vi "Agilent VNA Set External Trigger Mode.vi"(7 "Agilent VNA":T2, 8 "error in (no error)":errorcluster, 10 "Ext. Trigger Mode":T1, 11 "VISA Resource Name":refnum<visa-resource-name>) -> (0 "error out":errorcluster, 2 "Previous Ext. Trigger Mode":T1, 3 "dup VISA Resource Name":refnum<visa-resource-name>)   [LabVIEW 2011]
doc: "This VI for the HP8753B Network Analyzers reads the stimulus values. Except when performing log sweeps and freq list sweeps, this VI uses the start and stop values and the number of points to calcuate the stimulus values."
uses:
  TypeDefs/Agilent VNA External Trigger Mode.ctl
  TypeDefs/Agilent VNA Instrument Info.ctl
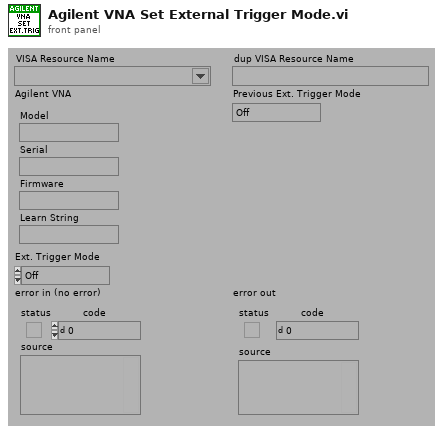
[diagram p1: front panel]
types:
  T1 = typedef "Agilent VNA External Trigger Mode.ctl" = enum16{"Off", "On Sweep", "On Point", "Manual On Point", "Internal", "External", "Bus"}
  T2 = typedef "Agilent VNA Instrument Info.ctl" = cluster{"Model":string, "Serial":string, "Firmware":string, "Learn String":string}
  T3 = typedef "Agilent VNA Model.ctl" = enum16{"Not Supported", "8510X", "8719X", "8720X", "8722X", "8753X", "ENA", "PNA", "Field Fox"}
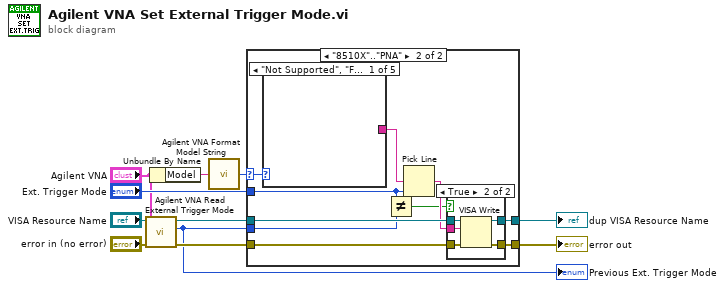
[diagram p0: block diagram]
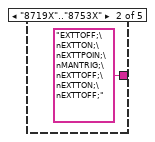
[diagram p3: hidden frame]
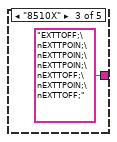
[diagram p4: hidden frame]
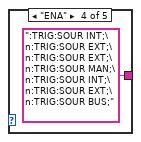
[diagram p5: hidden frame]
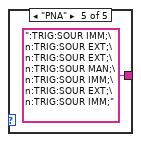
[diagram p6: hidden frame]
diagram:
  n1 = call "Agilent VNA Read External Trigger Mode.vi"("Agilent VNA"="Agilent VNA", "error in (no error)"="error in (no error)", "VISA Resource Name"="VISA Resource Name") -> ("error out"=w6:errorcluster, "Ext. Trigger Mode"=w4:T1, "dup VISA Resource Name"=w5:refnum<visa-resource-name>)  [unwired: 6 out]
  "Previous Ext. Trigger Mode" <- w4
  n2 = Unbundle By Name("Agilent VNA") -> ("Model"=w3:string)
  n3 = call "Agilent VNA Format Model String.vi"("Model"=w3) -> ("Model"=w1:T3)
  n4 = case shown="\"8510X\"..\"PNA\"" w1 {
    selector: w1 -> [_ w14]
    tunnel: [w13 w23] -> w11
    tunnel: [w12 w22] -> w10
    tunnel: "Ext. Trigger Mode" -> [_ w21]
    tunnel: w6 -> [w12 w20]
    tunnel: w5 -> [w13 w19]
    tunnel: w4 -> [_ w18]
    frame "Not Supported", "Field Fox" {
    }
    frame "8510X".."PNA" {
      n5 = case shown="\"Not Supported\", \"Field Fox\"" w14 {
        tunnel: [_ "EXTTOFF;\nEXTTON;\nEXTTPOIN;\nMANTRIG;\nEXTTOFF;\nEXTTON;\nEXTTOFF;" "EXTTOFF;\nEXTTPOIN;\nEXTTPOIN;\nEXTTPOIN;\nEXTTOFF;\nEXTTPOIN;\nEXTTOFF;" ":TRIG:SOUR INT;\n:TRIG:SOUR EXT;\n:TRIG:SOUR EXT;\n:TRIG:SOUR MAN;\n:TRIG:SOUR INT;\n:TRIG:SOUR EXT;\n:TRIG:SOUR BUS;" ":TRIG:SOUR IMM;\n:TRIG:SOUR EXT;\n:TRIG:SOUR EXT;\n:TRIG:SOUR MAN;\n:TRIG:SOUR IMM;\n:TRIG:SOUR EXT;\n:TRIG:SOUR IMM;"] -> w16
        frame "Not Supported", "Field Fox" {
        }
        frame "8719X".."8753X" {
        }
        frame "8510X" {
        }
        frame "ENA" {
        }
        frame "PNA" {
        }
      }
      n6 = Not Equal?(x=w21, y=w18) -> (x != y?=w15:bool)
      n7 = Pick Line(multi-line string=w16, line index=w21) -> (output string=w17:string)  [unwired: 1 out]
      n8 = case shown="True" w15 {
        tunnel: w20 -> [w28 w34]
        tunnel: w19 -> [w29 w33]
        tunnel: w17 -> [_ w32]
        tunnel: [w29 w31] -> w23
        tunnel: [w28 w30] -> w22
        frame False {
        }
        frame True {
          n9 = VISA Write(VISA resource name=w33, write buffer=w32, error in (no error)=w34) -> (VISA resource name out=w31:refnum<visa-resource-name>, error out=w30:errorcluster)  [unwired: 1 out]
        }
      }
    }
  }
  "dup VISA Resource Name" <- w11
  "error out" <- w10
